vi "Main.vi"(8 "Error In":errorcluster) -> (0 "Error Out":errorcluster)   [LabVIEW 2017, in "Scope.lvlib" / "Trigger.lvlib"]
uses:
  Trigger.lvlib
  Controls/Params.ctl
  Controls/Mode.ctl
  Controls/Trigger channels.ctl
  System Control/Main controller.lvlib
  Events/Events.lvlib
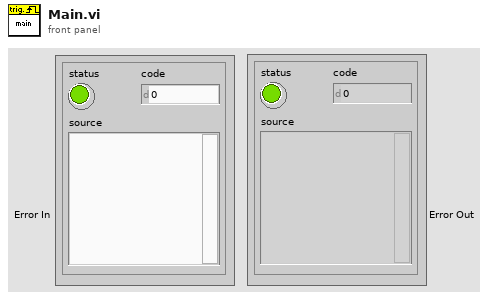
[diagram p1: front panel]
types:
  T1 = typedef "Scope.lvlib/Trigger.lvlib/Params.ctl" = cluster{"Mode":T2, "Source ":T3, "PIA mode":cluster{"Test LEDs":bool, "LED line":tag, "LED off (s)":dbl, "LED on (s)":dbl}, "Threshold (V)":dbl}
  T2 = typedef "Scope.lvlib/Trigger.lvlib/Mode.ctl" = enum32{"Laser (TAS)", "LED (PIA/VIA)"}
  T3 = typedef "Scope.lvlib/Trigger.lvlib/Trigger channels.ctl" = enum16{"Channel 1", "Channel 2", "Channel 3", "Channel 4", "AC Line", "Aux", "Digital Channel 0", "Digital Channel 1", "Digital Channel 2", "Digital Channel 3", "Digital Channel 4", "Digital Channel 5", "Digital Channel 6", "Digital Channel 7", "Digital Channel 8", "Digital Channel 9", "Digital Channel 10", "Digital Channel 11", "Digital Channel 12", "Digital Channel 13", "Digital Channel 14", "Digital Channel 15", "RF"}
  T4 = typedef "Events.lvlib/Refs [cluster].ctl" = cluster{"Exit":refnum<user-event>, "Controller":refnum<user-event>, "System Error":refnum<user-event>, "UI":refnum<user-event>, "Example Module":refnum<user-event>, "Shutter":refnum<user-event>, "Monochromator":refnum<user-event>, "DAQ":refnum<user-event>, "Scope":refnum<user-event>, "Processing":refnum<user-event>, "File IO":refnum<user-event>, "Colour wheel":refnum<user-event>}
  T5 = typedef "Example Module.lvlib/Commands [enum].ctl" = enum16{"Start", "Stop", "Send config"}
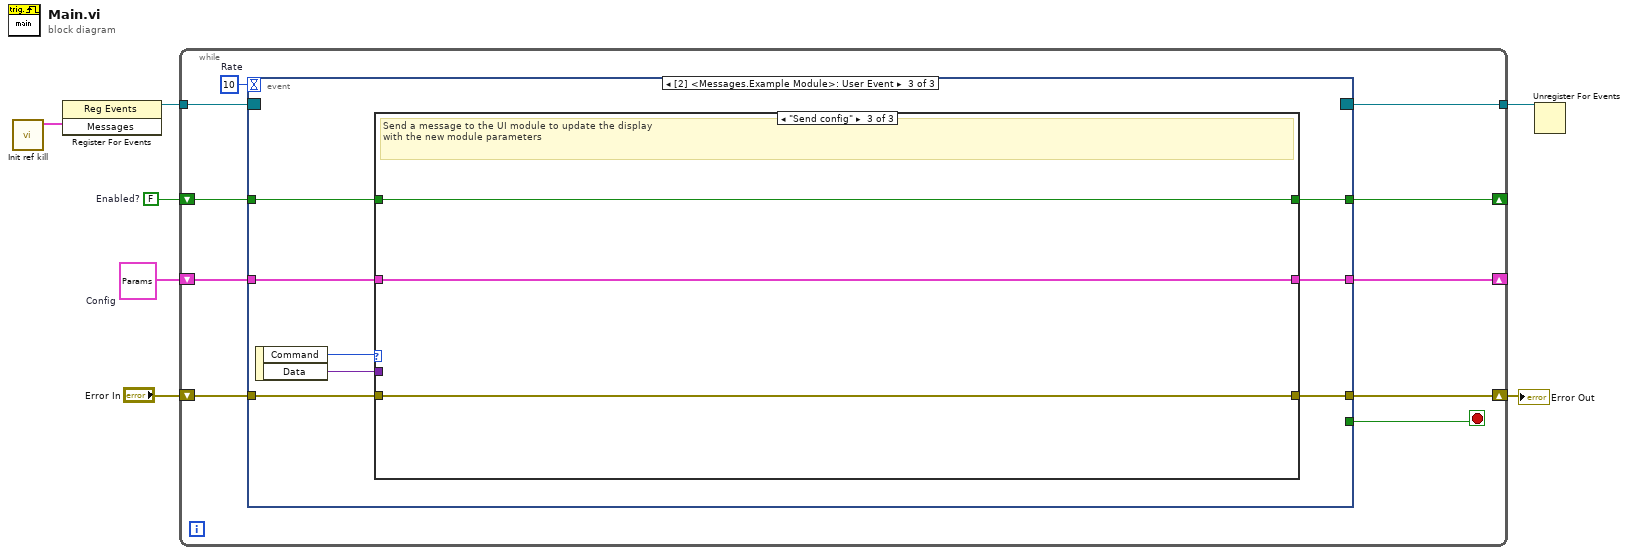
[diagram p0: block diagram]
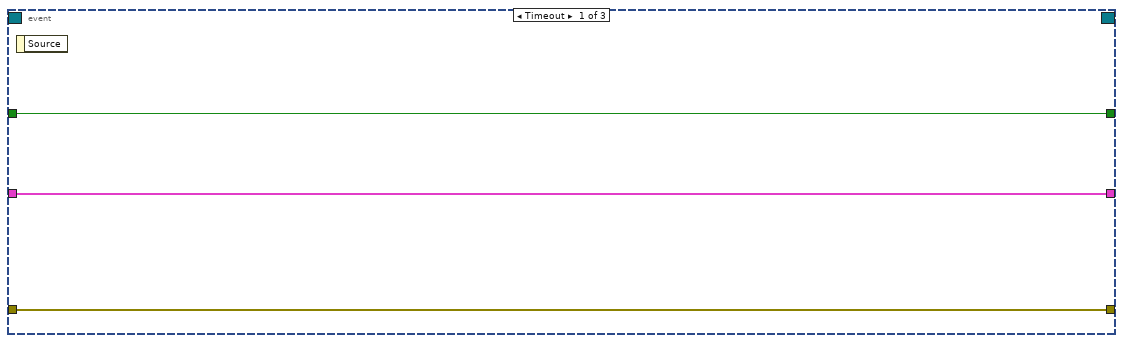
[diagram p2: hidden frame]
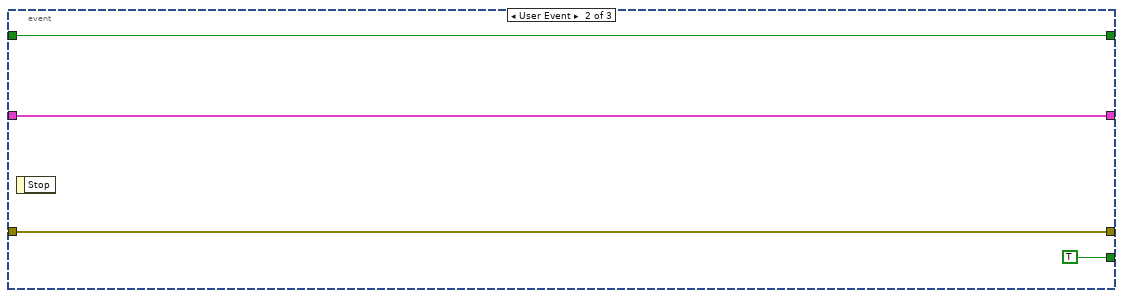
[diagram p3: hidden frame]
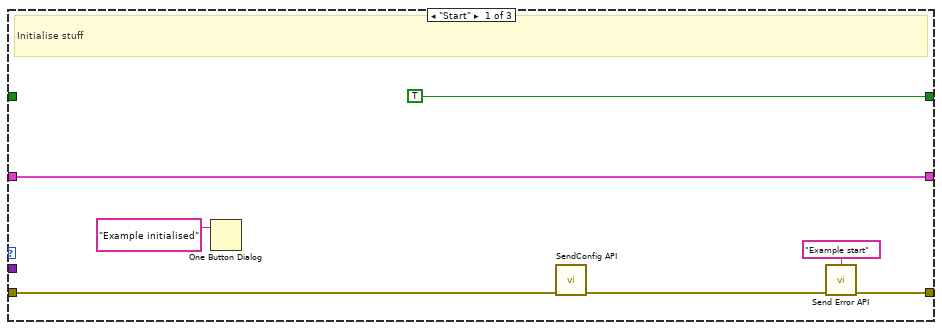
[diagram p4: hidden frame]
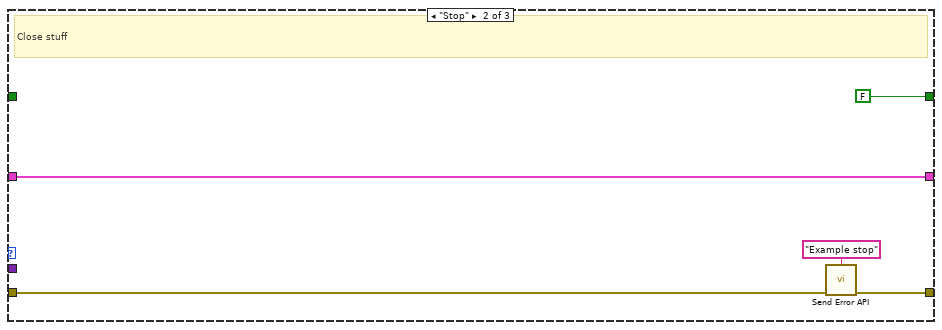
[diagram p5: hidden frame]
diagram:
  w1 = T1 {"Mode"=enum."Laser (TAS)", "Source "=enum."Channel 1", "PIA mode"={"Test LEDs"=FALSE, "LED line"="", "LED off (s)"=0.0, "LED on (s)"=0.0}, "Threshold (V)"=0.0}  # Config
  w5 = FALSE  # Enabled?
  n1 = call "Init ref kill.vi"() -> ("Messages"=w7:T4)  [unwired: 10 in, 1 out]
  n2 = register-events(w7) -> (reference out=w6:refnum<event-registration>)  [unwired: 2 in, 1 out]
  n3 = while {
    tunnel: w6 -> [w17]
    shift-right: [w13] -> _
    shift-left: w5 -> [w12]
    tunnel: [w14] -> w4
    shift-right: [w8] -> w2
    shift-left: "Error In" -> [w11]
    shift-right: [w9] -> _
    shift-left: w1 -> [w10]
    stop <- w15 stop-if-true
    w16 = 10  # Rate
    n4 = event shown="[2] <Messages.Example Module>: User Event" {
      selector: w17 -> [_ _ _]
      dyn-events: [_ _ _] -> w14
      timeout: w16 -> [_ _ _]
      tunnel: [_ TRUE _] -> w15
      tunnel: [w18 w21 w31] -> w13
      tunnel: w12 -> [w18 w21 w30]
      tunnel: w11 -> [w19 w22 w28]
      tunnel: [w19 w22 w27] -> w8
      tunnel: w10 -> [w20 w23 w26]
      tunnel: [w20 w23 w25] -> w9
      event Timeout {
        n5 = event-data() -> ()  [unwired: 1 in, 1 out]
      }
      event User Event {
        n6 = event-data() -> ()  [unwired: 1 in, 1 out]
      }
      event User Event {
        n7 = event-data() -> ("Command"=w32:T5, "Data"=w29:variant)  [unwired: 1 in]
        n8 = case shown="\"Send config\"" w32 {
          tunnel: [TRUE FALSE w46] -> w31
          tunnel: w30 -> [_ _ w46]
          tunnel: w29 -> [_ _ _]
          tunnel: w28 -> [w33 w40 w45]
          tunnel: [w37 w42 w45] -> w27
          tunnel: w26 -> [w34 w43 w47]
          tunnel: [w34 w43 w47] -> w25
          frame "Start" {
            # "Initialise stuff"
            n9 = One Button Dialog(message="Example initialised") -> ()  [unwired: 1 in, 1 out]
            n10 = call "SendConfig API.vi"("Error In"=w33) -> ("Error Out"=w38:errorcluster)  [unwired: 10 in]
            n11 = call "Send Error API.vi"("Error Cluster"=w38, "Error"="Example start") -> ("Error Out"=w37:errorcluster)  [unwired: 9 in]
          }
          frame "Stop" {
            # "Close stuff"
            n12 = call "Send Error API.vi"("Error Cluster"=w40, "Error"="Example stop") -> ("Error Out"=w42:errorcluster)  [unwired: 9 in]
          }
          frame "Send config" {
            # "Send a message to the UI module to update the display \nwith the new module parameters"
          }
        }
      }
    }
  }
  "Error Out" <- w2
  n13 = Unregister For Events(event registration refnum=w4) -> ()  [unwired: 1 in, 1 out]
